vi "CMD_03_Set_DAC1and2.vi"(8 "Input2, V":dbl min=-10.0 max=10.0, 9 "Input1, V":dbl min=-50.0 max=50.0, 11 "VISA resource name":refnum<visa-resource-name>) -> (3 "VISA resource name out":refnum<visa-resource-name>)   [LabVIEW 2017]
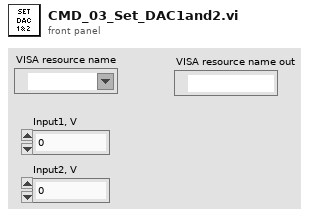
[diagram p1: front panel]
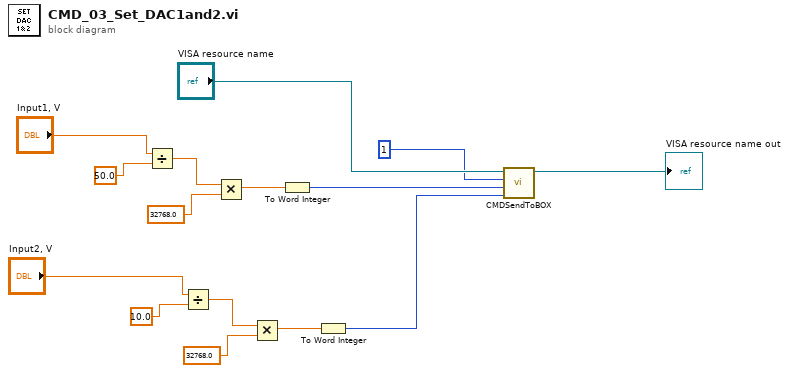
[diagram p0: block diagram]
diagram:
  n1 = Divide(x="Input1, V", y=50.0) -> (x/y=w12:dbl)
  n2 = Divide(x="Input2, V", y=10.0) -> (x/y=w5:dbl)
  n3 = Multiply(x=w12, y=32768.0) -> (x*y=w13:dbl)
  n4 = Multiply(x=w5, y=32768.0) -> (x*y=w6:dbl)
  n5 = To Word Integer(number=w13) -> (16bit integer=w8:i16)
  n6 = To Word Integer(number=w6) -> (16bit integer=w2:i16)
  n7 = call "CMDSendToBOX.vi"("arg2"=w2, "arg1"=w8, "CMD"=i8 1, "VISA resource name"="VISA resource name") -> ("VISA resource name out"=→"VISA resource name out":refnum<visa-resource-name>)  [unwired: 7 in]
